vi "InWindow3D.vi"(1 "Jitter":dbl, 2 "Radius":dbl=0.1, 3 "TargXYZ":dbl[](array[numeric])=[0.0, 0.0, 0.0], 4 "PosXYZ":dbl[](array[numeric])=[0.0, 0.0, 0.0]) -> (0 "Status":enum16{"In", "Out"}(ring)=enum."Out")   [LabVIEW 2013]
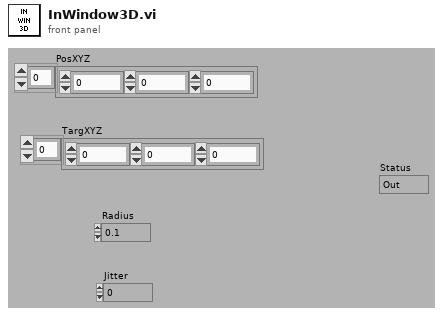
[diagram p1: front panel]
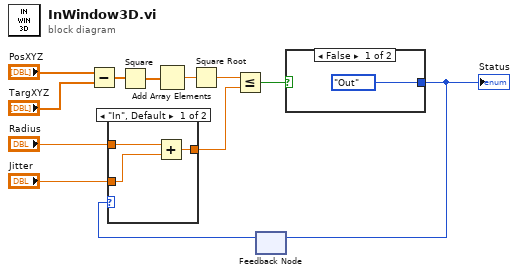
[diagram p0: block diagram]
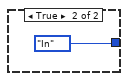
[diagram p3: hidden frame]
diagram:
  n1 = Subtract(x="PosXYZ", y="TargXYZ") -> (x-y=w6:dbl[])
  n2 = Square(x=w6) -> (x^2=w5:dbl[])
  n3 = Add Array Elements(numeric array=w5) -> (sum=w4:dbl)
  n4 = Square Root(x=w4) -> (sqrt(x)=w3:dbl)
  n5 = feedback #1() -> (w10:enum16{"In", "Out"})  [unwired: 1 in]
  n6 = case shown="\"In\", Default" w10 {
    tunnel: [w15 w16] -> w11
    tunnel: "Radius" -> [w14 w16]
    tunnel: "Jitter" -> [w13 _]
    frame "In", Default {
      n7 = Add(x=w14, y=w13) -> (x+y=w15:dbl)
    }
    frame "Out" {
    }
  }
  n8 = Less Or Equal?(x=w3, y=w11) -> (x <= y?=w12:bool)
  n9 = case shown="False" w12 {
    tunnel: [enum16{"In", "Out"}."Out" ("Fix.Status") enum16{"In", "Out"}."In" ("Fix.Status")] -> w9
    frame False {
    }
    frame True {
    }
  }
  "Status" <- w9
  n10 = feedback-in #1(w9) -> ()
